vi "Wire.vi"(8 "error in":errorcluster, 11 "reference":refnum<vi>) -> (0 "error out":errorcluster, 3 "wire":refnum<class "Wire.lvclass">)   [LabVIEW 2014, in "Raspberry Pi Compatible Compiler for LabVIEW.lvlib" / "Wire.lvclass"]
uses:
  Wire.lvclass
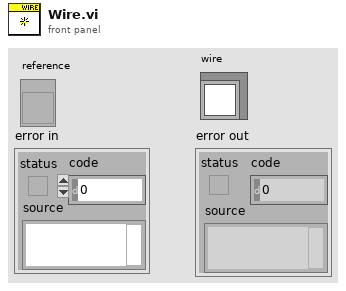
[diagram p1: front panel]
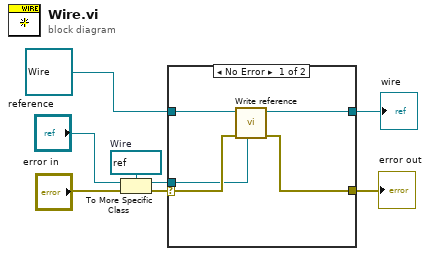
[diagram p0: block diagram]
diagram:
  w6 = refnum<vi> refnum  # Wire
  n1 = To More Specific Class(target class=w6, reference="reference", error in="error in") -> (specific class reference=w4:refnum<vi>, error out=w5:errorcluster)
  n2 = case shown="No Error" w5 {
    selector: w5 -> [w13 w15]
    tunnel: w4 -> [w11 _]
    tunnel: refnum<class "Wire.lvclass"> refnum ("Wire.lvclass") -> [w12 w14]
    tunnel: [w10 w14] -> w1
    tunnel: [w9 w15] -> w2
    frame No Error {
      n3 = call-dynamic "Write reference.vi"("reference"=w11, "error in"=w13, "GObject in"=w12) -> ("error out"=w9:errorcluster, "GObject out"=w10:refnum<class "Wire.lvclass">)  [unwired: 5 in]
    }
    frame Error {
    }
  }
  "error out" <- w2
  "wire" <- w1
